vi "VCS Open SubDevice Dlg.vi"(8 "error in (no error)":errorcluster, 11 "deviceHandle":u32) -> (0 "error out":errorcluster, 3 "keyHandle":u32)   [LabVIEW 2019, in "maxonEPOS.lvlib"]
doc: "<B>VCS Open SubDevice Dlg</B> recognizes available subdevices capable to operate with gateway device and opens the selected device for communication."
uses:
  Examples/maxonEPOS.lvlib
  Resources/EposCmd.dll
  Resources/EposCmd64.dll
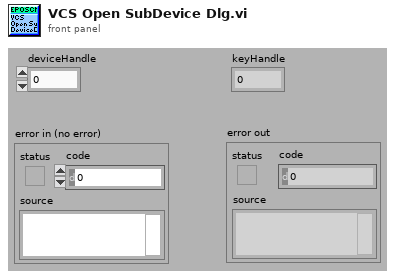
[diagram p1: front panel]
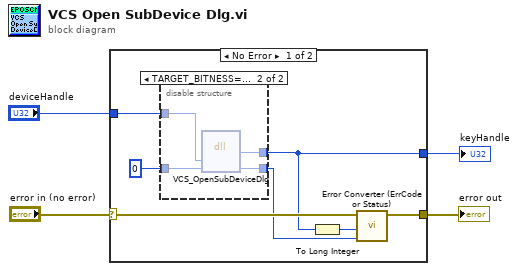
[diagram p0: block diagram]
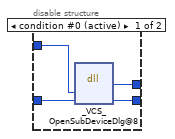
[diagram p2: hidden frame]
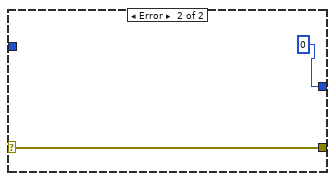
[diagram p3: hidden frame]
diagram:
  n1 = case shown="No Error" "error in (no error)" {
    selector: "error in (no error)" -> [w11 w21]
    tunnel: [w7 w21] -> w3
    tunnel: [w6 u32 0] -> w2
    tunnel: "deviceHandle" -> [w5 _]
    frame No Error {
      n2 = disable-structure shown="TARGET_BITNESS==64" {
        disable-tunnel: [w15 w19] -> w10
        disable-tunnel: u32 0 ("pErrorCode") -> [w14 w18]
        disable-tunnel: [w13 w17] -> w6
        disable-tunnel: w5 -> [w12 w16]
        frame condition #0 (active) {
          n3 = dll-call lib="C:/workspace/project/scancon/sw/SSI_Tool/InstrumentsInterfaces/Motordriver/maxon EPOS/Resources/EposCmd.dll" fn="_VCS_OpenSubDeviceDlg@8"("deviceHandle"=w12, "pErrorCode"=w14) -> ("keyHandle"=w13:u32, "pErrorCode"=w15:u32)  [unwired: 4 in, 2 out]
        }
        frame condition #1 {
          n4 = dll-call lib="C:/Sources/LabView/maxon EPOS/Resources/EposCmd64.dll" fn="VCS_OpenSubDeviceDlg"("deviceHandle"=w16, "pErrorCode"=w18) -> ("return type"=w17:u32, "pErrorCode"=w19:u32)  [unwired: 4 in, 2 out]
        }
      }
      n5 = To Long Integer(number=w6) -> (32bit integer=w8:i32)
      n6 = call "Error Converter (ErrCode or Status).vi"("error code"=w10, "return type"=w8, "error in (no error)"=w11) -> ("error out"=w7:errorcluster)  [unwired: 7 in]
    }
    frame Error {
    }
  }
  "error out" <- w3
  "keyHandle" <- w2
